vi "Reader Name to Reader List Item.vi"(3 "Reader Name":string) -> (0 "Reader List Item Integer":u16, 1 "Reader List Item":T1=enum."DAQmx Analog")   [LabVIEW 2017, in "Scan Driver.lvclass"]
uses:
  Scan Driver.lvclass
  Reader List.ctl
  <vilib>/Utility/error.llb/DialogType.ctl
panel:
  in  "Reader List.ctl":T1=enum."DAQmx Analog"
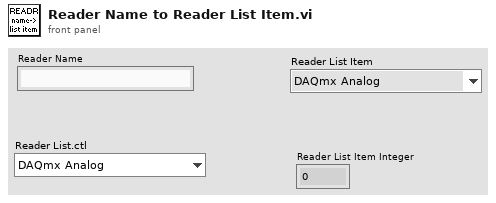
[diagram p1: front panel]
types:
  T1 = typedef "Scan Driver.lvclass/Reader List.ctl" = enum16{"Dummy", "Cryostat Temperature", "DAQmx Analog", "Lockin SR830", "Multimeter", "Photon Counter", "Power Meter", "Temperature Control"}
  T2 = typedef "DialogType.ctl" = u16
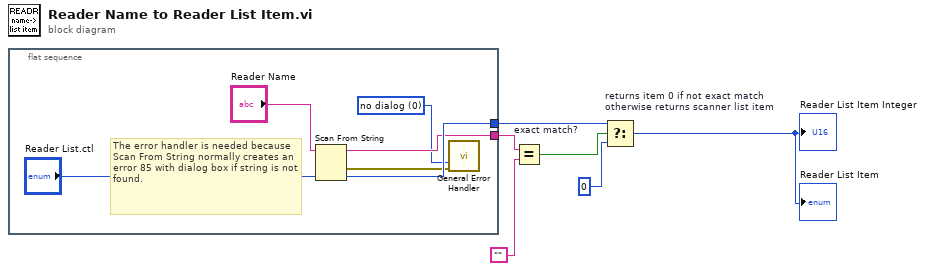
[diagram p0: block diagram]
diagram:
  n1 = flat-sequence {
    tunnel: [w12] -> w5
    tunnel: [w11] -> w3
    frame #0 {
      w8 = T2 0 items=["no dialog", "OK message", "continue or stop message", "OK message + warnings", "continue/stop + warnings"] ("type of dialog (OK msg:1)")
      # "The error handler is needed because Scan From String normally creates an error 85 with dialog box if string is not found."
      n2 = Scan From String "Scan From String"(input string="Reader Name", default 1="Reader List.ctl") -> (remaining string=w11:string, error out=w10:errorcluster, output 1=w12:T1)  [unwired: 3 in, 1 out]
      n3 = call <vilib>:"General Error Handler.vi"("type of dialog (OK msg:1)"=w8, "error in (no error)"=w10) -> ()  [unwired: 9 in, 5 out]
    }
  }
  n4 = Equal? "exact match?"(x=w3, y="") -> (x = y?=w4:bool)
  n5 = Select "returns item 0 if not exact match\notherwise returns scanner list item"(t=w5, s=w4, f=u16 0) -> (s? t:f=→"Reader List Item Integer" →"Reader List Item":u16)
